vi "Max Panels.vi"(8 "error in (no error)":errorcluster, 11 "SubPanel Grid View in":refnum<class "SubPanel Grid View.lvclass">) -> (0 "error out":errorcluster, 1 "Max Panels":i32, 3 "SubPanel Grid View out":refnum<class "SubPanel Grid View.lvclass">)   [LabVIEW 2012, in "Win8uiDemo.lvlib" / "SubPanel Grid View.lvclass"]
uses:
  SubPanel Grid View.lvclass
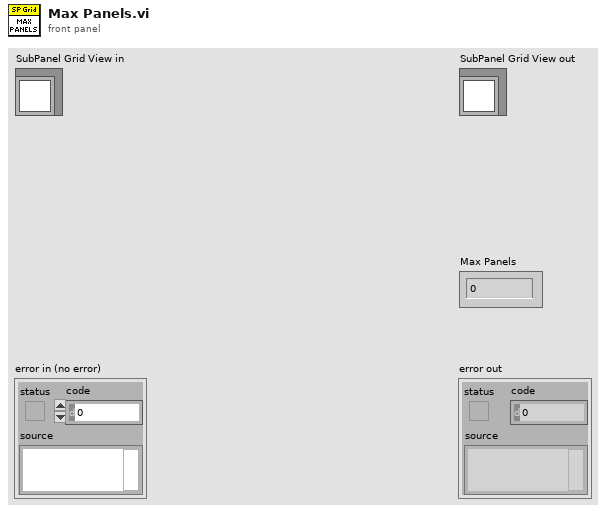
[diagram p1: front panel]
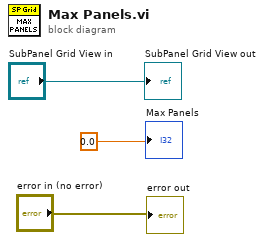
[diagram p0: block diagram]
diagram:
  "error out" <- "error in (no error)"
  "SubPanel Grid View out" <- "SubPanel Grid View in"
  "Max Panels" <- 0.0 ("Max Panels")
